vi "Set to unused all items right of last selected.vi"(8 "error in (no error)":errorcluster, 11 "Pool in":T1[](array[typedef])=[{"index"=0, "state"=enum."unused"}, {"index"=1, "state"=enum."unused"}, {"index"=2, "state"=enum."unused"}, {"index"=3, "state"=enum."unused"}, {"index"=4, "state"=enum."unused"}, {"index"=5, "state"=enum."unused"}]) -> (0 "error out":errorcluster, 3 "Pool out":T1[](array[typedef])=[{"index"=0, "state"=enum."unused"}, {"index"=1, "state"=enum."unused"}, {"index"=2, "state"=enum."unused"}, {"index"=3, "state"=enum."unused"}, {"index"=4, "state"=enum."unused"}, {"index"=5, "state"=enum."unused"}])   [LabVIEW 2021, in "Numeric Utilities.lvlib"]
uses:
  Numeric Utilities.lvlib
  cluster-touched index.ctl
  index state enum.ctl
panel:
  # "Development\ncontrols/indicators useful for development and testing, but which are not outputs of the VI"
  # "Input\nInputs to the VI"
  # "Output\nOutputs of the VI"
  # "Description\n\nBlank VI with error handling case. \n\nSummarize the use of this VI in this space."
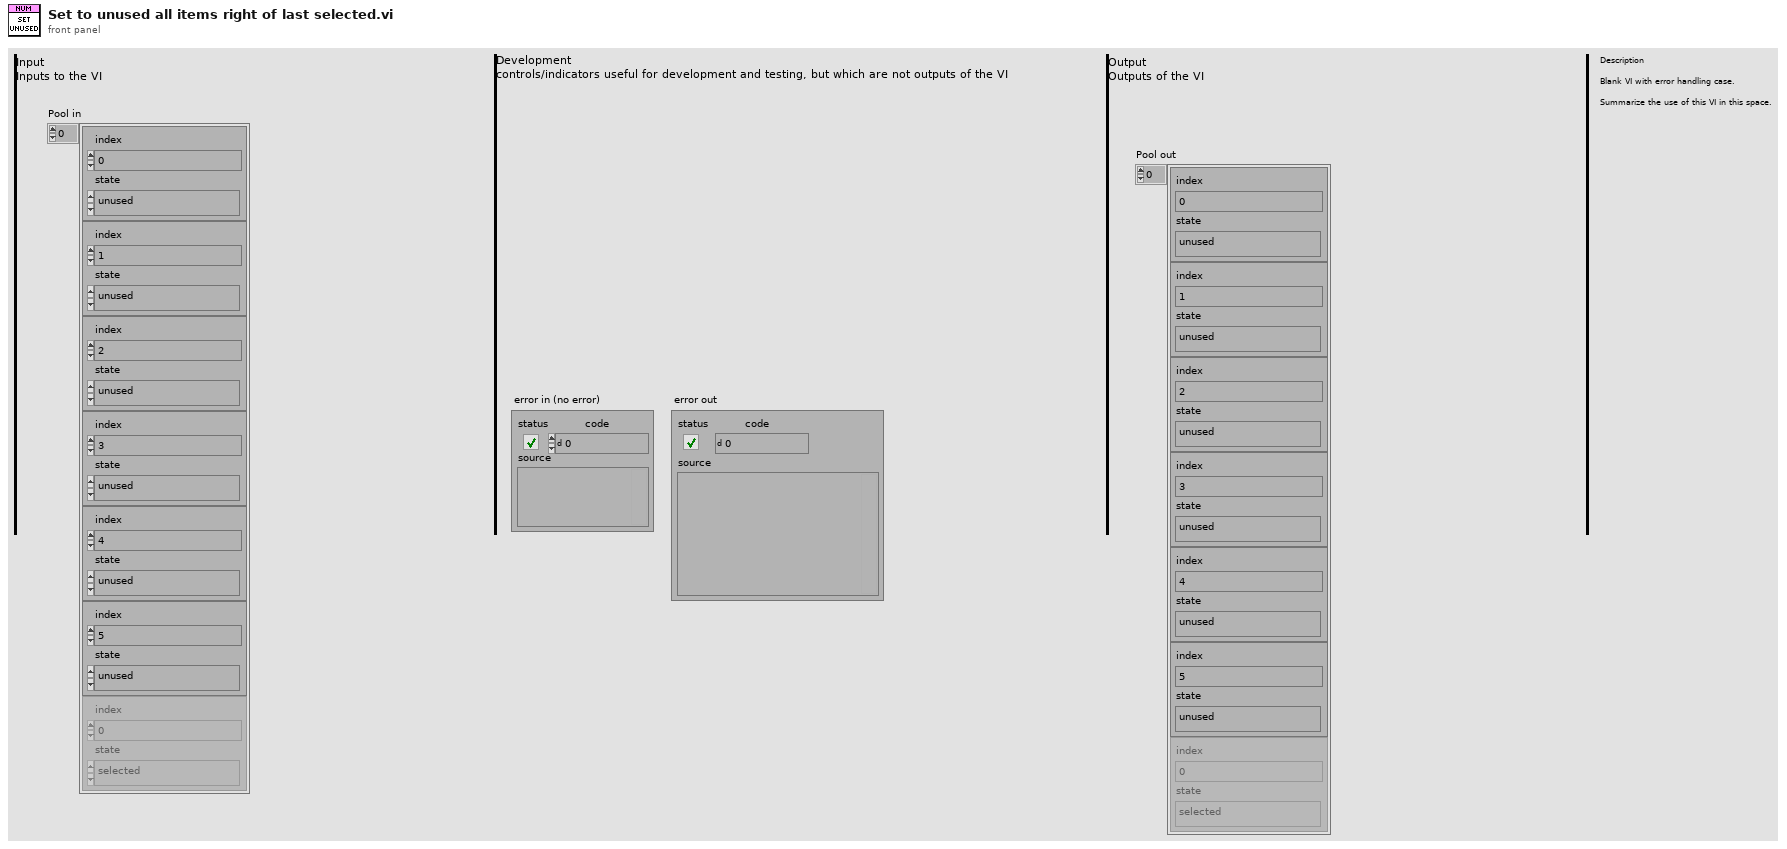
[diagram p1: front panel]
types:
  T1 = typedef "Numeric Utilities.lvlib/cluster-touched index.ctl" = cluster{"index":i32, "state":T2}
  T2 = typedef "Numeric Utilities.lvlib/index state enum.ctl" = enum16{"unused", "selected", "exhausted"}
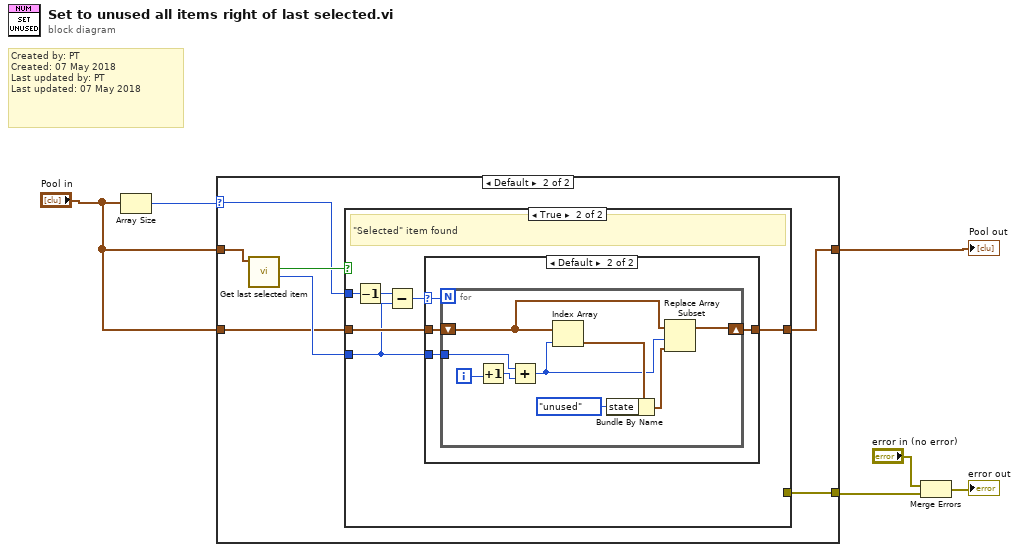
[diagram p0: block diagram]
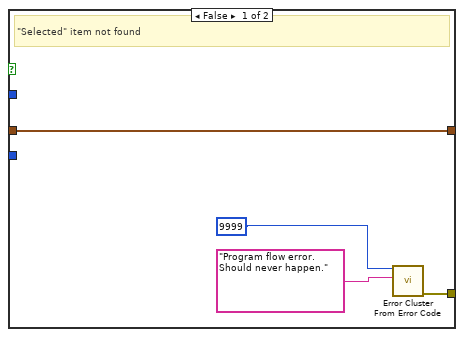
[diagram p3: hidden frame]
diagram:
  # "Created by: PT\nCreated: 07 May 2018\nLast updated by: PT\nLast updated: 07 May 2018"
  n1 = Array Size(array="Pool in") -> (size(s)=w6:i32)
  n2 = case shown="Default" w6 {
    selector: w6 -> [_ w8]
    tunnel: "Pool in" -> [w7 w14]
    tunnel: [w7 w9] -> w5
    tunnel: [_ w12] -> w2
    tunnel: "Pool in" -> [_ w10]
    frame 0 {
    }
    frame Default {
      n3 = call "Get last selected item.vi"("Pool"=w14) -> ("index of last selected item"=w11:i32, "T = selected item was found"=w13:bool)  [unwired: 7 in, 2 out]
      n4 = case shown="True" w13 {
        tunnel: [w17 _] -> w12
        tunnel: w11 -> [_ w20]
        tunnel: w10 -> [w15 w24]
        tunnel: [w15 w23] -> w9
        tunnel: w8 -> [_ w22]
        frame False {
          # "\"Selected\" item not found"
          n5 = call <vilib>:"Error Cluster From Error Code.vi"("error message (\"\")"="Program flow error. Should never happen.", "error code (0)"=9999) -> ("error out"=w17:errorcluster)  [unwired: 7 in]
        }
        frame True {
          # "\"Selected\" item found"
          n6 = Decrement(x=w22) -> (x-1=w21:i32)
          n7 = Subtract(x=w21, y=w20) -> (x-y=w19:i32)
          n8 = case shown="Default" w19 {
            selector: w19 -> [_ w26]
            tunnel: w24 -> [w25 w29]
            tunnel: [w25 w28] -> w23
            tunnel: w20 -> [_ w27]
            frame 0 {
            }
            frame Default {
              n9 = for {
                N: w26 -> [_]
                tunnel: w27 -> [w36]
                shift-right: [w30] -> w28
                shift-left: w29 -> [w33]
                i -> [w38]
                n10 = Increment(x=w38) -> (x+1=w37:i32)
                n11 = Add(x=w36, y=w37) -> (x+y=w31:i32)
                n12 = Index Array(array=w33, index=w31) -> (element=w35:T1)
                n13 = Bundle By Name(cluster=w35, "state"=index_state_enum."unused") -> (w32:T1)
                n14 = Replace Array Subset(array=w33, new element=w32, index=w31) -> (w30:T1[])
              }
            }
          }
        }
      }
    }
  }
  "Pool out" <- w5
  n15 = Merge Errors("error in (no error)", w2) -> (→"error out":errorcluster)
